vi "Demo.vi"(0 "LED Outputs":T3, 1 "VISA resource name":refnum<visa-resource-name>="COM5", 2 "stop":bool) -> (14 "Analog Inputs":T1, 15 "Switch Inputs":T2, 16 "Updates / Second":dbl, 17 "CRC Status":bool, 18 "CRC Failures":i32)   [LabVIEW 2013]
uses:
  LED_Output_TypeDef.ctl
  Switch_Input_TypeDef.ctl
  Analog_Input_TypeDef.ctl
  PWM_Output_TypeDef.ctl
panel:
  in  "data bits (8)":u16=8 min=5 max=8 step=1
  in  "Slide":u8(slide) scale=0.0..180.0
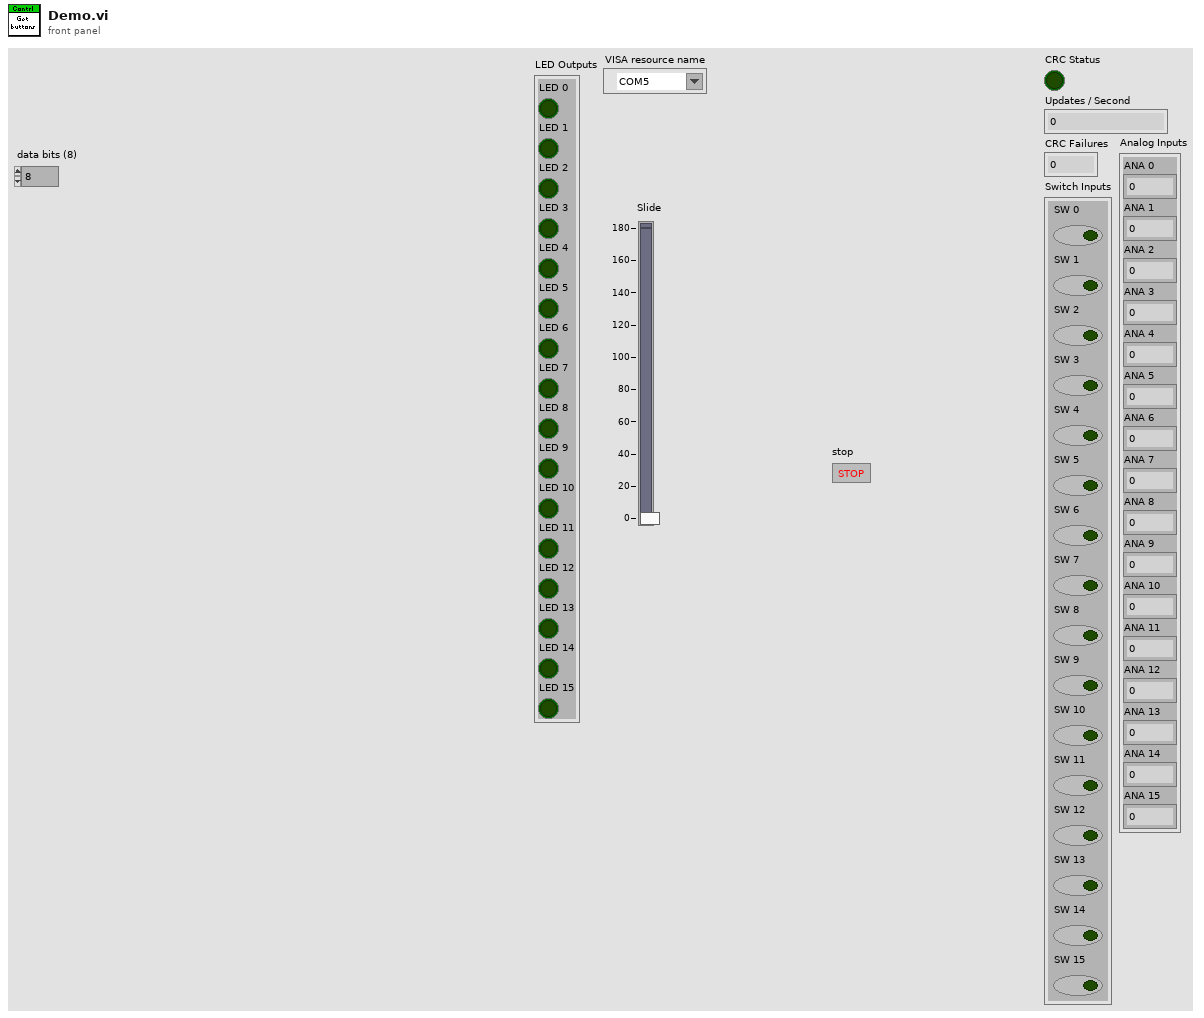
[diagram p1: front panel]
types:
  T1 = typedef "Analog_Input_TypeDef.ctl" = cluster{"ANA 0":u8, "ANA 1":u8, "ANA 2":u8, "ANA 3":u8, "ANA 4":u8, "ANA 5":u8, "ANA 6":u8, "ANA 7":u8, "ANA 8":u8, "ANA 9":u8, "ANA 10":u8, "ANA 11":u8, "ANA 12":u8, "ANA 13":u8, "ANA 14":u8, "ANA 15":u8}
  T2 = typedef "Switch_Input_TypeDef.ctl" = cluster{"SW 0":bool, "SW 1":bool, "SW 2":bool, "SW 3":bool, "SW 4":bool, "SW 5":bool, "SW 6":bool, "SW 7":bool, "SW 8":bool, "SW 9":bool, "SW 10":bool, "SW 11":bool, "SW 12":bool, "SW 13":bool, "SW 14":bool, "SW 15":bool}
  T3 = typedef "LED_Output_TypeDef.ctl" = cluster{"LED 0":bool, "LED 1":bool, "LED 2":bool, "LED 3":bool, "LED 4":bool, "LED 5":bool, "LED 6":bool, "LED 7":bool, "LED 8":bool, "LED 9":bool, "LED 10":bool, "LED 11":bool, "LED 12":bool, "LED 13":bool, "LED 14":bool, "LED 15":bool}
  T4 = typedef "PWM_Output_TypeDef.ctl" = cluster{"PWM 0":u8, "PWM 1":u8, "PWM 2":u8, "PWM 3":u8, "PWM 4":u8, "PWM 5":u8, "PWM 6":u8, "PWM 7":u8, "PWM 8":u8, "PWM 9":u8, "PWM 10":u8}
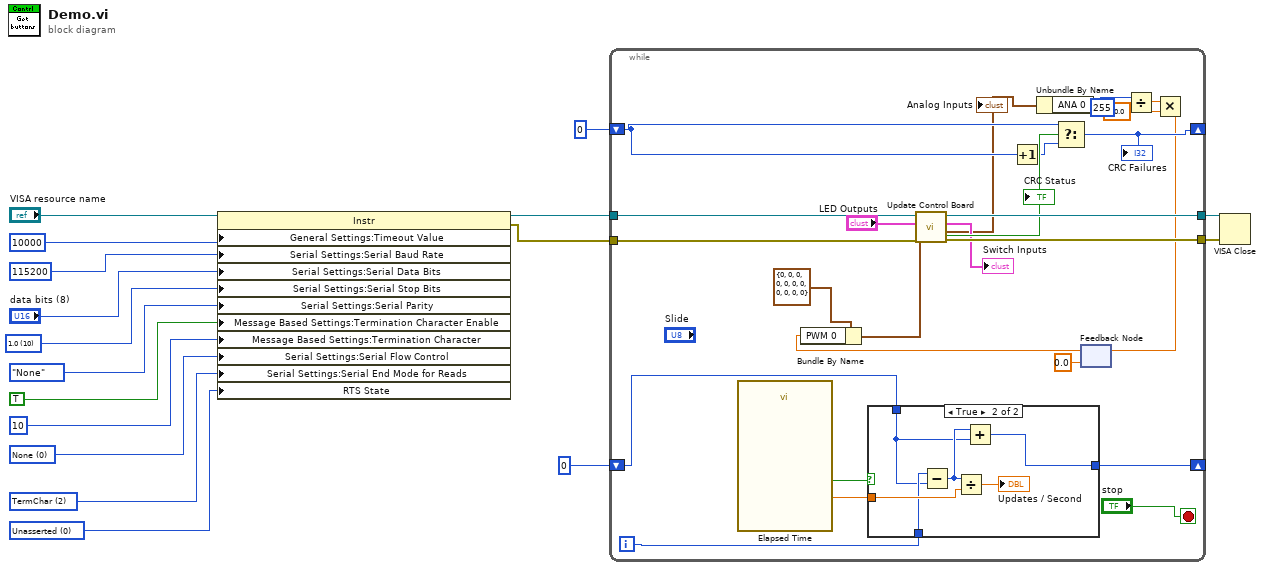
[diagram p0: block diagram]
diagram:
  w8 = u16 2 items=["None", "LastBit", "TermChar"] ("Serial Settings:Serial End Mode for Reads")
  w1 = i16 0 items=["Unknown"=-1, "Unasserted"=0, "Asserted"=1] ("Serial Settings:Modem Line Settings:Line RTS State")
  w6 = u16 0 items=["None", "XON/XOFF", "RTS/CTS", "XON/XOFF & RTS/CTS", "DTR/DSR", "XON/XOFF & DTR/DSR"] ("flow control (0:none)")
  w9 = u16 10 items=["1.0"=10, "1.5"=15, "2.0"=20] ("stop bits (10: 1 bit)")
  n1 = property class="Instr"(reference="VISA resource name", "General Settings:Timeout Value"=u32 10000 ("timeout (10sec)"), "Serial Settings:Serial Baud Rate"=u32 115200 ("baud rate (9600)"), "Serial Settings:Serial Data Bits"="data bits (8)", "Serial Settings:Serial Stop Bits"=w9, "Serial Settings:Serial Parity"=enum16{"None", "Odd", "Even", "Mark", "Space"}."None" ("parity (0:none)"), "Message Based Settings:Termination Character Enable"=TRUE ("Enable Termination\nChar (T)"), "Message Based Settings:Termination Character"=u8 10 ("termination char\n(0xA = '\\n' = LF)"), "Serial Settings:Serial Flow Control"=w6, "Serial Settings:Serial End Mode for Reads"=w8, "RTS State"=w1) -> (reference out=w5:refnum<visa-resource-name>, error out=w4:errorcluster)  [unwired: 1 in]
  n2 = while {
    tunnel: w5 -> [w42]
    tunnel: w4 -> [w41]
    tunnel: [w38] -> w17
    tunnel: [w37] -> w16
    shift-right: [w33] -> _
    shift-left: 0 -> [w34]
    shift-right: [w28] -> _
    shift-left: 0 -> [w29]
    i -> [w32]
    stop <- "stop" stop-if-true
    n3 = call "Elapsed Time"() -> ("Elapsed Time (s)"=w35:dbl, "Time has Elapsed"=w36:bool)  [unwired: 12 in, 6 out]
    n4 = case shown="True" w36 {
      tunnel: w35 -> [_ w50]
      tunnel: w34 -> [w44 w45]
      tunnel: [w44 w48] -> w33
      tunnel: w32 -> [_ w49]
      frame False {
      }
      frame True {
        n5 = Subtract(x=w49, y=w45) -> (x-y=w46:i32)
        n6 = Divide(x=w46, y=w50) -> (x/y=→"Updates / Second":dbl)
        n7 = Add(x=w46, y=w45) -> (x+y=w48:i32)
      }
    }
    n8 = Increment(x=w29) -> (x+1=w30:i32)
    n9 = feedback #1(0.0) -> (w19:dbl)
    n10 = Bundle By Name(cluster=T4 {"PWM 0"=0, "PWM 1"=0, "PWM 2"=0, "PWM 3"=0, "PWM 4"=0, "PWM 5"=0, "PWM 6"=0, "PWM 7"=0, "PWM 8"=0, "PWM 9"=0, "PWM 10"=0} ("PWM Outputs"), "PWM 0"=w19) -> (w39:T4)
    n11 = call "Update Control Board.vi"("error in (no error)"=w41, "PWM Outputs"=w39, "LED Outputs"="LED Outputs", "Control Board VISA Reference In"=w42) -> ("error out"=w38:errorcluster, "Analog Inputs"=w25:T1, "Switch Inputs"=→"Switch Inputs":T2, "Control Board VISA Reference Out"=w37:refnum<visa-resource-name>, "CRC Status"=w31:bool)  [unwired: 3 in]
    "CRC Status" <- w31
    "Analog Inputs" <- w25
    n12 = Unbundle By Name(w25) -> ("ANA 0"=w24:u8)
    n13 = Select(t=w29, s=w31, f=w30) -> (s? t:f=w28:i32)
    "CRC Failures" <- w28
    n14 = Divide(x=w24, y=u8 255) -> (x/y=w22:dbl)
    n15 = Multiply(x=w22, y=180.0) -> (x*y=w20:dbl)
    n16 = feedback-in #1(w20) -> ()
  }
  n17 = VISA Close(VISA resource name=w16, error in (no error)=w17) -> ()  [unwired: 1 out]
